vi "setUserEvents.vi"(10 "UserEvents":refnum<class "UserEvents.lvclass">, 11 "Telemetry in":refnum<class "Telemetry.lvclass">) -> (3 "Telemetry out":refnum<class "Telemetry.lvclass">)   [LabVIEW 2016, in "Telemetry.lvclass"]
uses:
  Telemetry.lvclass
  UserEvents/UserEvents.lvclass
  Telemetry.lvclass/Telemetry.ctl
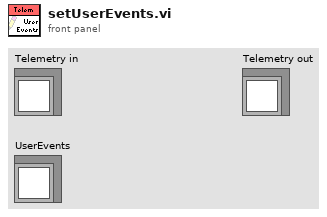
[diagram p1: front panel]
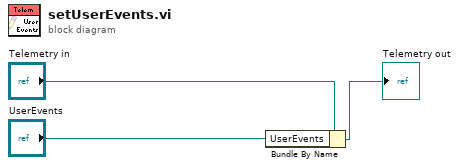
[diagram p0: block diagram]
diagram:
  n1 = Bundle By Name(cluster="Telemetry in", "UserEvents"="UserEvents") -> (→"Telemetry out":refnum<class "Telemetry.lvclass">)
